vi "PI Retrieve Key Array for Config.vi"(8 "error in (no error)":errorcluster, 10 "Key Array In":T7, 11 "Connection Refnum":T1) -> (0 "error out":errorcluster, 2 "Prompted Inputs Test Parameters":T2, 3 "Connection Refnum":T1)   [LabVIEW 2011]
uses:
  ITK EXT/utils/keyedarr.llb/Keyed Array.ctl
  TypeDefs/PI Test Parameters.ctl
  TypeDefs/PI Measurement Cluster.ctl
  TypeDefs/PI Limit Parameters.ctl
  TypeDefs/PI Limit Definition.ctl
  TypeDefs/PI Limit Comparison.ctl
  Summitek EXT/ODBC/SQL Controls/Connection Refnum.ctl
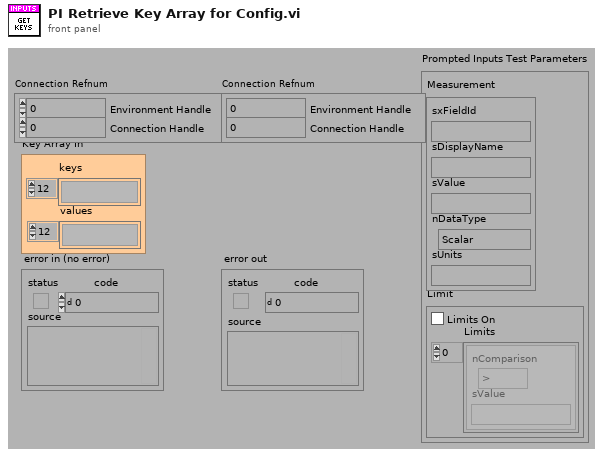
[diagram p1: front panel]
types:
  T1 = typedef "Connection Refnum.ctl" = cluster{"Environment Handle":i32, "Connection Handle":i32}
  T2 = typedef "PI Test Parameters.ctl" = cluster{"Measurement":T3, "Limit":T4}
  T3 = typedef "PI Measurement Cluster.ctl" = cluster{"sxFieldId":string, "sValue":string, "nDataType":enum16{"Scalar", "Enumeration"}, "sUnits":string, "sDisplayName":string}
  T4 = typedef "PI Limit Parameters.ctl" = cluster{"Limits On":bool, "Limits":T5[]}
  T5 = typedef "PI Limit Definition.ctl" = cluster{"nComparison":T6, "sValue":string}
  T6 = typedef "PI Limit Comparison.ctl" = enum16{">", ">=", "<", "<=", "<>", "="}
  T7 = typedef "Keyed Array.ctl" = cluster{"keys":string[], "values":string[]}
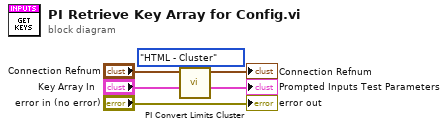
[diagram p0: block diagram]
diagram:
  n1 = call "PI Convert Limits Cluster.vi"("Conversion"=enum16{"Cluster - HTML", "HTML - Cluster"}."HTML - Cluster", "PI Key Array In"="Key Array In") -> ("PI Cluster Out"=→"Prompted Inputs Test Parameters":T2)  [unwired: 1 in, 6 out]
  "error out" <- "error in (no error)"
  "Connection Refnum" <- "Connection Refnum"
